vi "Register Test Channel View.vi"(11 "Message Enqueuer in":refnum<class "Message Enqueuer.lvclass">) -> (3 "Message Enqueuer out":refnum<class "Message Enqueuer.lvclass">)   [LabVIEW 2013]
uses:
  <vilib>/ActorFramework/Message Enqueuer/Message Enqueuer.lvclass
  <vilib>/ActorFrameworkMVC/View Observer/Registration Message/Registration Message.lvclass
  <vilib>/ActorFrameworkMVC/View Observer/Data Message/Data Message.lvclass
  Models/Test Channel Model Messages/Register Test Channel Move In Next Msg/Register Test Channel Move In Next Msg.lvclass
  Models/Test Channel Model Messages/Register Test Channel Move In Previous Msg/Register Test Channel Move In Previous Msg.lvclass
  Models/Test Channel Model Messages/Register Test Channel Next Button Visibility Msg/Register Test Channel Next Button Visibility Msg.lvclass
  Models/Test Channel Model Messages/Register Test Channel Previous Button Visibility Msg/Register Test Channel Previous Button Visibility Msg.lvclass
  Models/Test Channel Model Messages/Register Test Channel Tiles Info Msg/Register Test Channel Tiles Info Msg.lvclass
  Views/Test Channel View Messages/Conceret Test Channel Move In Next Msg/Conceret Test Channel Move In Next Msg.lvclass
  Views/Test Channel View Messages/Conceret Test Channel Move In Previous Msg/Conceret Test Channel Move In Previous Msg.lvclass
  Views/Test Channel View Messages/Conceret Test Channel Next Button Visibility Msg/Conceret Test Channel Next Button Visibility Msg.lvclass
  Views/Test Channel View Messages/Conceret Test Channel Previous Button Visibility Msg/Conceret Test Channel Previous Button Visibility Msg.lvclass
  Views/Test Channel View Messages/Conceret Test Channel Tiles Info Msg/Conceret Test Channel Tiles Info Msg.lvclass
  <vilib>/ActorFrameworkMVC/UI Controller Messages/Subscribe View to Model Msg/Subscribe View to Model Msg.lvclass/Subscribe View to Model Msg.ctl
  <vilib>/ActorFramework/Message Enqueuer/Message Enqueuer.lvclass/Message Enqueuer.ctl
  <vilib>/ActorFramework/Message Enqueuer/Enqueue.vi
  <vilib>/ActorFramework/Message Priority Queue/Priority Enqueue.vi
  <vilib>/ActorFrameworkMVC/UI Controller Messages/Subscribe View to Model Msg/Subscribe View to Model Msg.lvclass
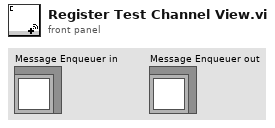
[diagram p1: front panel]
types:
  T1 = cluster{"Registration Message":string, "Data Message":string}[]
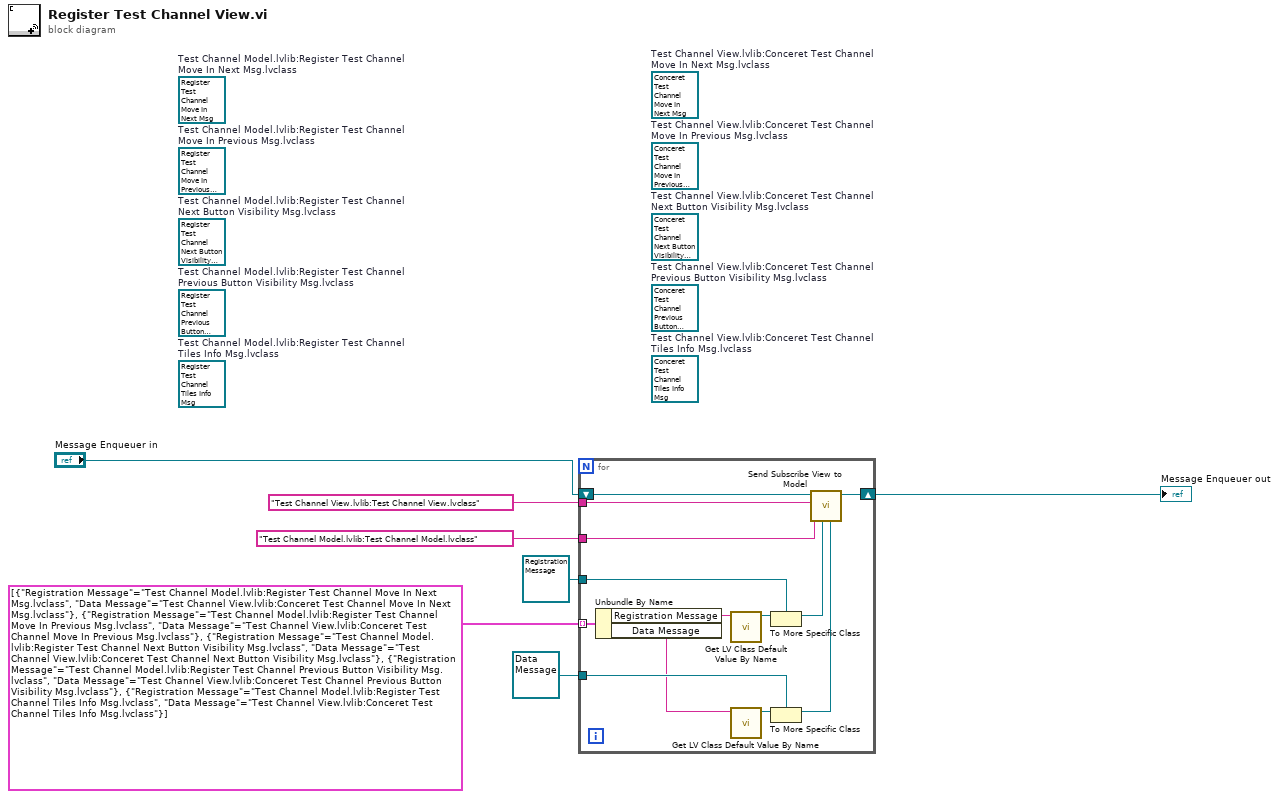
[diagram p0: block diagram]
diagram:
  (unwired) refnum<class "Conceret Test Channel Tiles Info Msg.lvclass"> refnum  # Test Channel View.lvlib:Conceret Test Channel Tiles Info Msg.lvclass
  (unwired) refnum<class "Conceret Test Channel Previous Button Visibility Msg.lvclass"> refnum  # Test Channel View.lvlib:Conceret Test Channel Previous Button Visibility Msg.lvclass
  (unwired) refnum<class "Conceret Test Channel Next Button Visibility Msg.lvclass"> refnum  # Test Channel View.lvlib:Conceret Test Channel Next Button Visibility Msg.lvclass
  (unwired) refnum<class "Conceret Test Channel Move In Previous Msg.lvclass"> refnum  # Test Channel View.lvlib:Conceret Test Channel Move In Previous Msg.lvclass
  (unwired) refnum<class "Conceret Test Channel Move In Next Msg.lvclass"> refnum  # Test Channel View.lvlib:Conceret Test Channel Move In Next Msg.lvclass
  (unwired) refnum<class "Register Test Channel Tiles Info Msg.lvclass"> refnum  # Test Channel Model.lvlib:Register Test Channel Tiles Info Msg.lvclass
  (unwired) refnum<class "Register Test Channel Previous Button Visibility Msg.lvclass"> refnum  # Test Channel Model.lvlib:Register Test Channel Previous Button Visibility Msg.lvclass
  (unwired) refnum<class "Register Test Channel Next Button Visibility Msg.lvclass"> refnum  # Test Channel Model.lvlib:Register Test Channel Next Button Visibility Msg.lvclass
  (unwired) refnum<class "Register Test Channel Move In Previous Msg.lvclass"> refnum  # Test Channel Model.lvlib:Register Test Channel Move In Previous Msg.lvclass
  (unwired) refnum<class "Register Test Channel Move In Next Msg.lvclass"> refnum  # Test Channel Model.lvlib:Register Test Channel Move In Next Msg.lvclass
  n1 = for {
    tunnel: "Test Channel View.lvlib:Test Channel View.lvclass" ("View Name") -> [w19]
    tunnel: "Test Channel Model.lvlib:Test Channel Model.lvclass" ("Model Name") -> [w18]
    shift-right: [w17] -> w7
    shift-left: "Message Enqueuer in" -> [w20]
    tunnel: refnum<class "Registration Message.lvclass"> refnum ("Registration Message") -> [w14]
    tunnel: refnum<class "Data Message.lvclass"> refnum ("Data Message") -> [w13]
    tunnel: T1 [{"Registration Message"="Test Channel Model.lvlib:Register Test Channel Move In Next Msg.lvclass", "Data Message"="Test Channel View.lvlib:Conceret Test Channel Move In Next Msg.lvclass"}, {"Registration Message"="Test Channel Model.lvlib:Register Test Channel Move In Previous Msg.lvclass", "Data Message"="Test Channel View.lvlib:Conceret Test Channel Move In Previous Msg.lvclass"}, {"Registration Message"="Test Channel Model.lvlib:Register Test Channel Next Button Visibility Msg.lvclass", "Data Message"="Test Channel View.lvlib:Conceret Test Channel Next Button Visibility Msg.lvclass"}, {"Registration Message"="Test Channel Model.lvlib:Register Test Channel Previous Button Visibility Msg.lvclass", "Data Message"="Test Channel View.lvlib:Conceret Test Channel Previous Button Visibility Msg.lvclass"}, {"Registration Message"="Test Channel Model.lvlib:Register Test Channel Tiles Info Msg.lvclass", "Data Message"="Test Channel View.lvlib:Conceret Test Channel Tiles Info Msg.lvclass"}] -> [w12] mode=indexing
    n2 = Unbundle By Name(w12) -> ("Registration Message"=w9:string, "Data Message"=w8:string)
    n3 = call <vilib>:"Get LV Class Default Value By Name.vi"("class name"=w9) -> ("object"=w16:refnum<class>)  [unwired: 9 in, 1 out]
    n4 = call <vilib>:"Get LV Class Default Value By Name.vi"("class name"=w8) -> ("object"=w15:refnum<class>)  [unwired: 9 in, 1 out]
    n5 = To More Specific Class(target class=w14, reference=w16) -> (specific class reference=w11:refnum<class "Registration Message.lvclass">)  [unwired: 1 in, 1 out]
    n6 = To More Specific Class(target class=w13, reference=w15) -> (specific class reference=w10:refnum<class "Data Message.lvclass">)  [unwired: 1 in, 1 out]
    n7 = call <vilib>:"Send Subscribe View to Model.vi"("Data Message"=w10, "Registration Message"=w11, "Model Name"=w18, "View Name"=w19, "Message Enqueuer"=w20) -> ("Message Enqueuer out"=w17:refnum<class "Message Enqueuer.lvclass">)  [unwired: 5 in, 1 out]
  }
  "Message Enqueuer out" <- w7
